vi "BB_Draw_rect.vi"(8 "Error In":errorcluster, 11 "Image In":T1) -> (0 "Error Out":errorcluster, 3 "Image":T1(plugin-control) caption="Camera Image")   [LabVIEW 2012]
uses:
  <vilib>/vision/Image Controls.llb/IMAQ Image.ctl
  <vilib>/vision/NI_Vision_Development_Module.lvlib
panel:
  in  "Error In 2":errorcluster
  in  "Start Point 2":cluster{"X":i32, "Y":i32}={"X"=295, "Y"=0}
  in  "Stop Point 2":cluster{"X":i32, "Y":i32}={"X"=283, "Y"=480}
  in  "Stop Point":cluster{"X":i32, "Y":i32}={"X"=640, "Y"=272}
  in  "Start Point":cluster{"X":i32, "Y":i32}={"X"=23, "Y"=0}
  in  "Image Source":enum32{"File Images", "Live Camera"}(ring)=enum."Live Camera"
  in  "File List":i32(listbox)
  in  "Directory":path
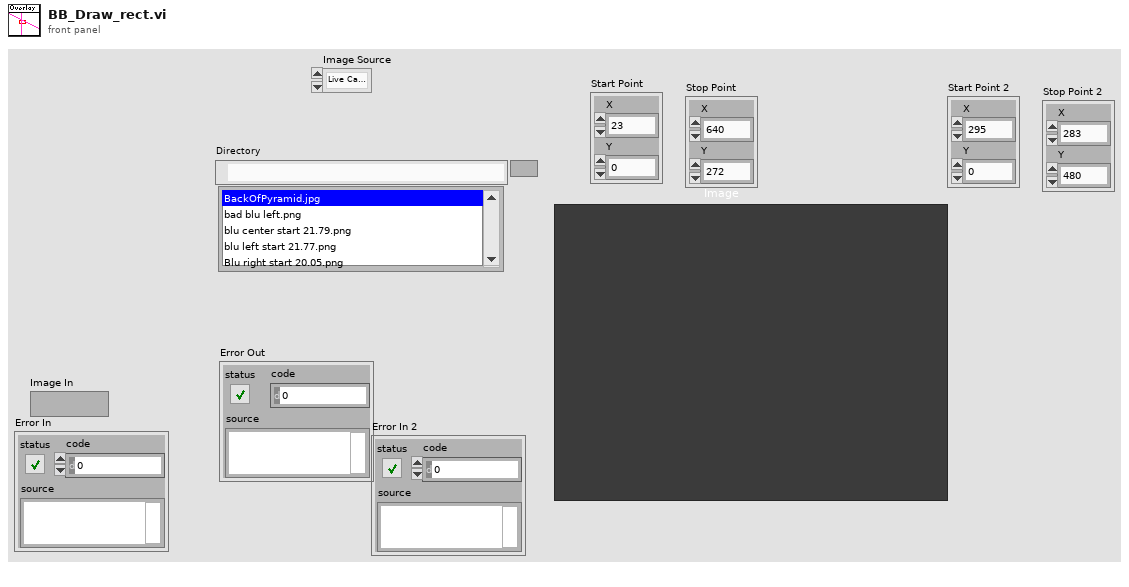
[diagram p1: front panel]
types:
  T1 = typedef "IMAQ Image.ctl" = refnum<image>
  T2 = typedef "Image Type" = u32
  T3 = cluster{"Left":i32, "Top":i32, "Right":i32, "Bottom":i32}
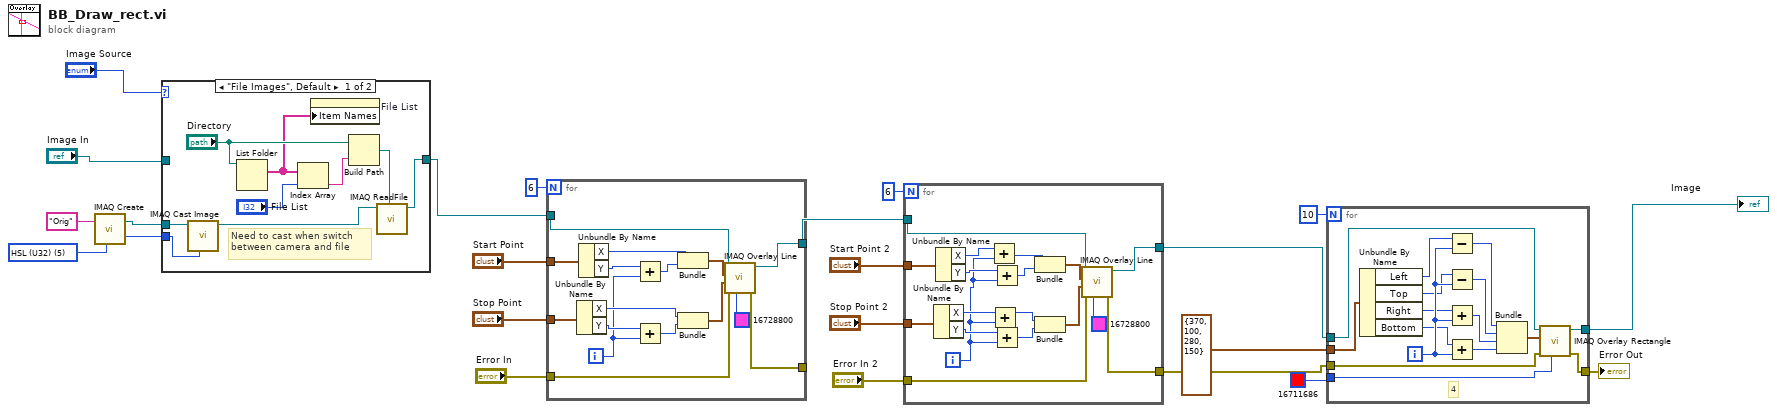
[diagram p0: block diagram]
diagram:
  w16 = T2 5 items=["Grayscale (U8)", "Grayscale (I16)", "Grayscale (SGL)", "Complex (CSG)", "RGB (U32)", "HSL (U32)", "RGB (U64)", "Grayscale (U16)"] ("Image Type")
  n1 = call "IMAQ Create"("Image Name"="Orig", "Image Type"=w16) -> ("New Image"=w15:T1)  [unwired: 2 in, 2 out]
  n2 = case shown="\"File Images\", Default" "Image Source" {
    tunnel: [w25 w32] -> w12
    tunnel: "Image In" -> [_ w32]
    tunnel: w16 -> [w24 _]
    tunnel: w15 -> [w23 _]
    frame "File Images", Default {
      # "Need to cast when switch\nbetween camera and file"
      n3 = call "IMAQ Cast Image"("Image Type"=w24, "Image Src"=w23) -> ("Image Dst Out"=w26:T1)  [unwired: 8 in, 1 out]
      n4 = List Folder(path="Directory") -> (filenames=w27:string[])  [unwired: 3 in, 3 out]
      n5 = Index Array(array=w27, index="File List") -> (element=w30:string)
      n6 = property on="File List" class="LstBox (strict)"("Item Names"=w27) -> ()  [unwired: 2 in, 2 out]
      n7 = Build Path(base path="Directory", name or relative path=w30) -> (appended path=w29:path)
      n8 = call "IMAQ ReadFile"("File Path"=w29, "Image"=w26) -> ("Image Out"=w25:T1)  [unwired: 5 in, 4 out]
    }
    frame "Live Camera" {
    }
  }
  n9 = for {
    N: 6 -> [_]
    tunnel: w12 -> [w48]
    tunnel: [w47] -> w3
    tunnel: "Start Point" -> [w43]
    tunnel: "Stop Point" -> [w42]
    tunnel: "Error In" -> [w46]
    tunnel: [w45] -> _
    i -> [w33]
    n10 = Unbundle By Name(w42) -> ("X"=w36:i32, "Y"=w34:i32)
    n11 = Unbundle By Name(w43) -> ("X"=w39:i32, "Y"=w37:i32)
    n12 = Add(x=w37, y=w33) -> (x+y=w38:i32)
    n13 = Add(x=w34, y=w33) -> (x+y=w35:i32)
    n14 = Bundle("X"=w39, w38) -> (w41:cluster{"X":i32, i32})  [unwired: 1 in]
    n15 = Bundle("X"=w36, w35) -> (w40:cluster{"X":i32, i32})  [unwired: 1 in]
    n16 = call "IMAQ Overlay Line"("Color"=u32 16728800, "error in (no error)"=w46, "End Point"=w40, "Start Point"=w41, "Image"=w48) -> ("error out"=w45:errorcluster, "Image Out"=w47:T1)  [unwired: 5 in]
  }
  n17 = for {
    N: 6 -> [_]
    tunnel: w3 -> [w66]
    tunnel: [w65] -> w2
    tunnel: "Start Point 2" -> [w61]
    tunnel: "Stop Point 2" -> [w60]
    tunnel: "Error In 2" -> [w64]
    tunnel: [w63] -> w1
    i -> [w49]
    n18 = Unbundle By Name(w60) -> ("X"=w54:i32, "Y"=w52:i32)
    n19 = Unbundle By Name(w61) -> ("X"=w57:i32, "Y"=w55:i32)
    n20 = Add(x=w57, y=w49) -> (x+y=w51:i32)
    n21 = Add(x=w54, y=w49) -> (x+y=w50:i32)
    n22 = Add(x=w55, y=w49) -> (x+y=w56:i32)
    n23 = Add(x=w52, y=w49) -> (x+y=w53:i32)
    n24 = Bundle(w51, w56) -> (w59:cluster{i32, i32})  [unwired: 1 in]
    n25 = Bundle(w50, w53) -> (w58:cluster{i32, i32})  [unwired: 1 in]
    n26 = call "IMAQ Overlay Line"("Color"=u32 16728800, "error in (no error)"=w64, "End Point"=w58, "Start Point"=w59, "Image"=w66) -> ("error out"=w63:errorcluster, "Image Out"=w65:T1)  [unwired: 5 in]
  }
  n27 = for {
    N: 10 -> [_]
    tunnel: w2 -> [w82]
    tunnel: w1 -> [w81]
    tunnel: [w80] -> w13
    tunnel: T3 {"Left"=370, "Top"=100, "Right"=280, "Bottom"=150} ("Rectangle") -> [w79]
    tunnel: u32 16711686 ("Color") -> [w68]
    tunnel: [w67] -> w20
    i -> [w78]
    # "4"
    n28 = Unbundle By Name(w79) -> ("Left"=w77:i32, "Top"=w76:i32, "Right"=w74:i32, "Bottom"=w75:i32)
    n29 = Subtract(x=w77, y=w78) -> (x-y=w73:i32)
    n30 = Subtract(x=w76, y=w78) -> (x-y=w72:i32)
    n31 = Add(x=w74, y=w78) -> (x+y=w71:i32)
    n32 = Add(x=w75, y=w78) -> (x+y=w70:i32)
    n33 = Bundle(w73, w72, w71, w70) -> (w69:cluster{i32, i32, i32, i32})  [unwired: 1 in]
    n34 = call "IMAQ Overlay Rectangle"("Color"=w68, "error in (no error)"=w81, "Rectangle"=w69, "Image"=w82) -> ("error out"=w67:errorcluster, "Image Out"=w80:T1)  [unwired: 6 in]
  }
  "Error Out" <- w20
  "Image" <- w13
